vi "test Create Messages Single Routing Channel Change State.vi"(8 "error in (no error)":errorcluster, 11 "TestCase in":refnum<class "Routing and Faulting Create Messages Unit Tests.lvclass">) -> (0 "error out":errorcluster, 3 "TestCase out":refnum<class "Routing and Faulting Create Messages Unit Tests.lvclass">)   [LabVIEW 2020, in "Routing and Faulting Create Messages Unit Tests.lvclass"]
uses:
  Routing and Faulting Create Messages Unit Tests.lvclass
  Engine/Engine Data.ctl
  Shared/Compiled.Settings.ctl
  Shared/Communication Configuration.ctl
  Shared/Routing and Faulting Configuration.ctl
  Shared/Routing Channel Configuration.ctl
  Shared/Value-Connections Map.ctl
  Shared/Alias Mapping.ctl
  Shared/Alias Endpoint.ctl
  Shared/Compiled Connection.ctl
  Shared/FIFO Indices.ctl
  Includes/CDMessaging.lvlibp/Producer/Abstract Producer/Abstract Producer.lvclass
  Engine/Device Inputs.ctl
  Engine/Device Outputs.ctl
  Includes/CDMessaging.lvlibp/Switch/Switch Connect Message/Switch Connect Message.lvclass
  C:/Users/mjacobso/Desktop/SCM/Routing-Faulting/Includes/CDMessaging.lvlibp/Message/Abstract Message/Abstract Message.lvclass
  Engine/Producer Message.ctl
  Includes/CDMessaging.lvlibp/Message/Abstract Message/Abstract Message.lvclass
  <vilib>/addons/_JKI Toolkits/VI Tester/TestCase.llb/TestCase.lvclass
  Engine/Routing and Faulting Engine.lvlib
  Shared/Routing and Faulting Shared.lvlib
  C:/Program Files (x86)/National Instruments/LabVIEW 2020/vi.lib/addons/_JKI Toolkits/VI Tester/TestCase.llb/TestCase.lvclass
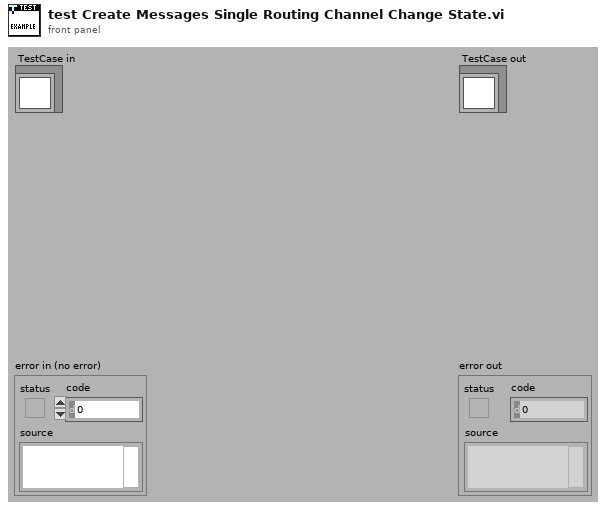
[diagram p1: front panel]
types:
  T1 = typedef "Routing and Faulting Shared.lvlib/Routing Channel Configuration.ctl" = cluster{"Channel Name":string, "Initial Value":dbl, "FIFO Index":i32, "Value-Connections Map":T2}
  T2 = typedef "Routing and Faulting Shared.lvlib/Value-Connections Map.ctl" = cluster{"State Value Array":i32[], "Connection List Array":cluster{"Compiled Connections Indices":i32[]}[]}
  T3 = typedef "Routing and Faulting Shared.lvlib/Compiled Connection.ctl" = cluster{"Consumer Queue Index":i32, "Normalized Connection String":string}
  T4 = typedef "Routing and Faulting Engine.lvlib/Producer Message.ctl" = cluster{"Consumer":string, "Message":refnum<class "Abstract Message.lvclass">}
  T5 = typedef "Routing and Faulting Shared.lvlib/Communication Configuration.ctl" = cluster{"Consumer Queue Names":string[]}
  T6 = typedef "Routing and Faulting Shared.lvlib/Routing and Faulting Configuration.ctl" = cluster{"Routing Channel Configurations":T1[], "Alias Mappings":T7[], "Compiled Connection Buffer":T3[], "Compiled Initial Connection Indices":i32[]}
  T7 = typedef "Routing and Faulting Shared.lvlib/Alias Mapping.ctl" = cluster{"Alias":string, "Endpoint":T8}
  T8 = typedef "Routing and Faulting Shared.lvlib/Alias Endpoint.ctl" = cluster{"Module Path":string, "Endpoint":string}
  T9 = typedef "Routing and Faulting Engine.lvlib/Engine Data.ctl" = cluster{"Compiled.Settings":T10, "Producer":refnum<class "Abstract Producer.lvclass">, "Device Inputs":T12, "Device Outputs":T13, "States Changed":bool[]}
  T10 = typedef "Routing and Faulting Shared.lvlib/Compiled.Settings.ctl" = cluster{"Custom Device Name":string, "Communication Configuration":T5, "Routing and Faulting Configuration":T6, "Status Channels FIFO Indices":T11}
  T11 = typedef "Routing and Faulting Shared.lvlib/FIFO Indices.ctl" = cluster{"Status Channel":i32, "Heartbeat Channel":i32}
  T12 = typedef "Routing and Faulting Engine.lvlib/Device Inputs.ctl" = cluster{"Current Inputs":dbl[], "Previous Inputs":dbl[], "Device Inputs FIFO":refnum<k33>}
  T13 = typedef "Routing and Faulting Engine.lvlib/Device Outputs.ctl" = cluster{"Outputs":dbl[], "Device Outputs FIFO":refnum<k33>}
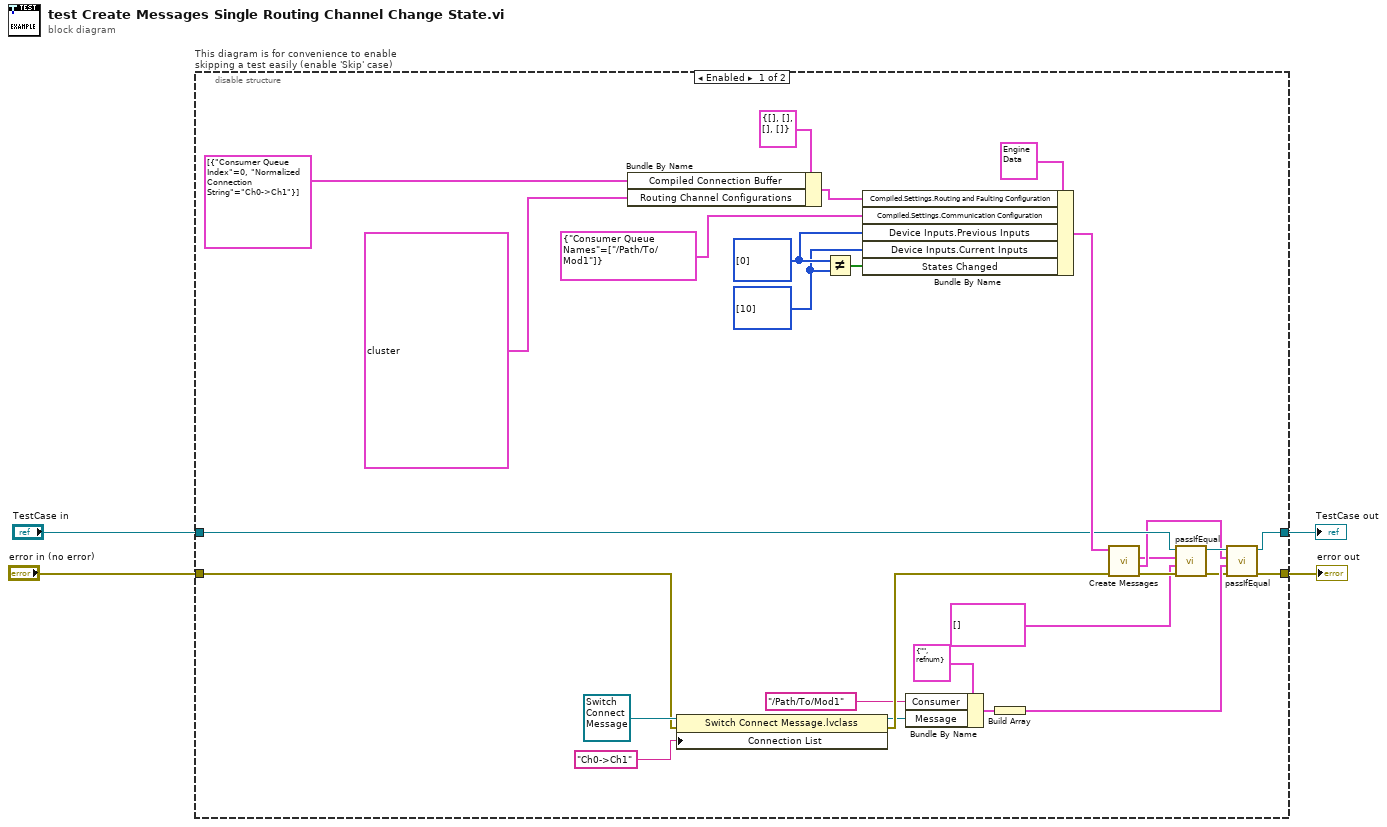
[diagram p0: block diagram]
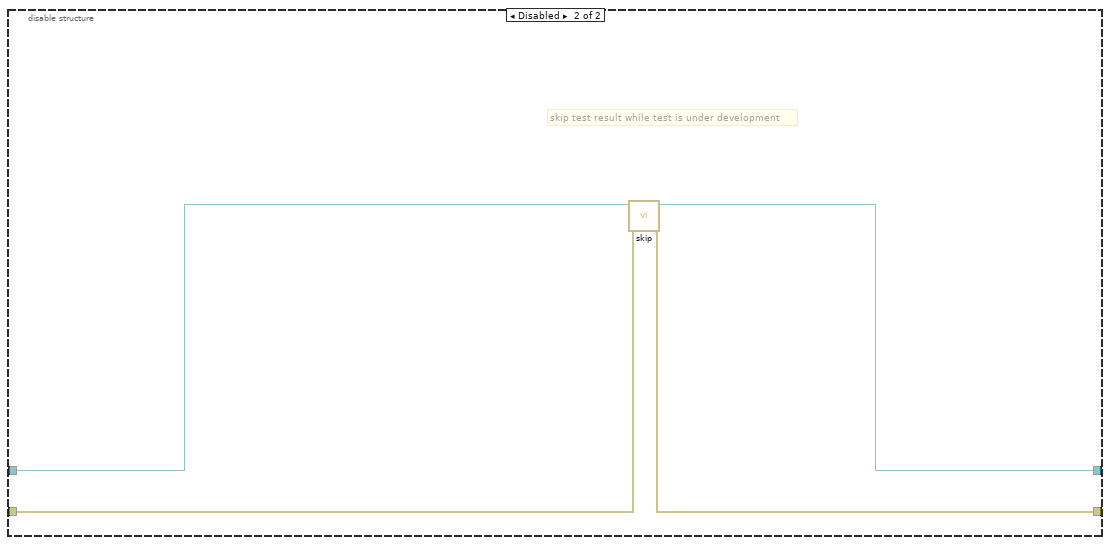
[diagram p2: hidden frame]
diagram:
  n1 = disable-structure "This diagram is for convenience to enable skipping a test easily (enable 'Skip' case)" shown="Enabled" {
    disable-tunnel: "TestCase in" -> [w10 w36]
    disable-tunnel: [w23 w34] -> w1
    disable-tunnel: [w24 w35] -> w3
    disable-tunnel: "error in (no error)" -> [w21 w33]
    frame Enabled {
      w28 = i32[] [10] ("State Value Array")
      w29 = i32[] [0] ("State Value Array")
      n2 = Bundle By Name(cluster=T6 {"Routing Channel Configurations"=[], "Alias Mappings"=[], "Compiled Connection Buffer"=[], "Compiled Initial Connection Indices"=[]} ("Compiled.Settings.Routing and Faulting Configuration"), "Compiled Connection Buffer"=T3[] [{"Consumer Queue Index"=0, "Normalized Connection String"="Ch0->Ch1"}], "Routing Channel Configurations"=T1[] [{"Channel Name"="Window Up", "Initial Value"=0.0, "FIFO Index"=0, "Value-Connections Map"={"State Value Array"=[0, 10], "Connection List Array"=[{"Compiled Connections Indices"=[]}, {"Compiled Connections Indices"=[0]}]}}]) -> (w30:T6)
      n3 = property class="Switch Connect Message.lvclass"(reference=refnum<class "Switch Connect Message.lvclass"> refnum ("CDMessaging.lvlibp:Switch Connect Message.lvclass"), error in=w21, "Connection List"="Ch0->Ch1") -> (reference out=w18:refnum<class "Switch Connect Message.lvclass">, error out=w20:errorcluster)
      n4 = Not Equal?(x=w29, y=w28) -> (x != y?=w27:bool[])
      n5 = Bundle By Name(cluster=T9 {"Compiled.Settings"={"Custom Device Name"="", "Communication Configuration"={"Consumer Queue Names"=[]}, "Routing and Faulting Configuration"={"Routing Channel Configurations"=[], "Alias Mappings"=[], "Compiled Connection Buffer"=[], "Compiled Initial Connection Indices"=[]}, "Status Channels FIFO Indices"={"Status Channel"=0, "Heartbeat Channel"=0}}, "Producer"=refnum, "Device Inputs"={"Current Inputs"=[], "Previous Inputs"=[], "Device Inputs FIFO"=refnum}, "Device Outputs"={"Outputs"=[], "Device Outputs FIFO"=refnum}, "States Changed"=[]} ("Engine Data in"), "Compiled.Settings.Routing and Faulting Configuration"=w30, "Compiled.Settings.Communication Configuration"=T5 {"Consumer Queue Names"=["/Path/To/Mod1"]}, "Device Inputs.Previous Inputs"=w29, "Device Inputs.Current Inputs"=w28, "States Changed"=w27) -> (w25:T9)
      n6 = Bundle By Name(cluster=T4 {"Consumer"="", "Message"=refnum} ("Producer Message"), "Consumer"="/Path/To/Mod1", "Message"=w18) -> (w16:T4)
      n7 = Build Array(w16) -> (w15:T4[])
      n8 = call "Create Messages.vi"("error in (no error)"=w20, "Engine Data in"=w25) -> ("error out"=w13:errorcluster, "Connect Messages"=w9:T4[], "Disconnect Messages"=w8:T4[])  [unwired: 6 in, 1 out]
      n9 = call-dynamic "passIfEqual.vi"("error in (no error)"=w13, "y"=T4[] [] ("Array"), "x"=w8, "TestCase in"=w10) -> ("error out"=w12:errorcluster, "TestCase out"=w11:refnum<class "Routing and Faulting Create Messages Unit Tests.lvclass">)  [unwired: 6 in]
      n10 = call-dynamic "passIfEqual.vi"("error in (no error)"=w12, "y"=w15, "x"=w9, "TestCase in"=w11) -> ("error out"=w24:errorcluster, "TestCase out"=w23:refnum<class "Routing and Faulting Create Messages Unit Tests.lvclass">)  [unwired: 6 in]
    }
    frame Disabled {
      # "skip test result while test is under development"
      n11 = call <vilib>:"skip.vi"("error in (no error)"=w33, "TestCase in"=w36) -> ("error out"=w35:errorcluster, "TestCase out"=w34:refnum<class "Routing and Faulting Create Messages Unit Tests.lvclass">)  [unwired: 8 in]
    }
  }
  "error out" <- w3
  "TestCase out" <- w1
